vi "Log In.vi"(0 "session in":refnum<k21>, 1 "username":string, 2 "password":string, 5 "chassis":refnum<k21>, 11 "error in (no error)":errorcluster, 12 "connect timeout (60 sec)":dbl=60.0, 13 "save credentials to disk? (F)":bool) -> (4 "session out":refnum<k21>, 15 "error out":errorcluster)   [LabVIEW 2020, in "SLSC.lvlib"]
doc: "Saves login credentials for an SLSC chassis on the local system. When the SLSC driver opens a network connection to an SLSC chassis, it checks whether there are any saved login credentials for this chassis. If so, the SLSC driver uses the saved login credentials. Otherwise, the SLSC driver tries default credentials with anonymous as the username and an empty string as the password."
uses:
  <vilib>/SLSC/SLSC.lvlib
  nislsclvapi.dll
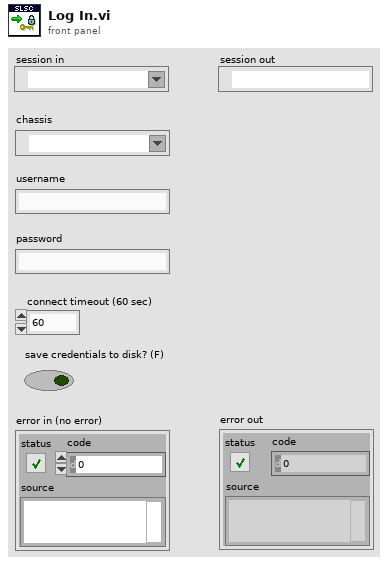
[diagram p1: front panel]
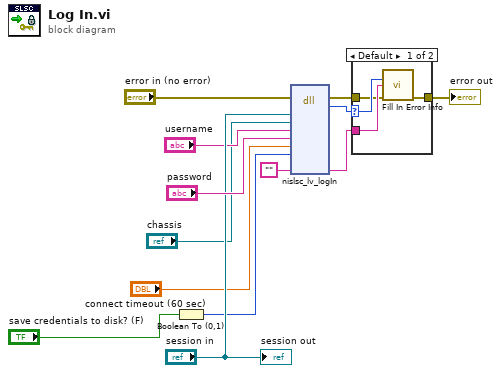
[diagram p0: block diagram]
diagram:
  n1 = Boolean To (0,1)(Boolean="save credentials to disk? (F)") -> (0, 1=w1:i16)
  n2 = dll-call lib="nislsclvapi.*" fn="nislsc_lv_logIn"(error in="error in (no error)", "session"="session in", "chassis"="chassis", "username"="username", "password"="password", "timeout"="connect timeout (60 sec)", "saveCredentialsToDisk"=w1, "extendedErrorInfo"="") -> (error out=w9:errorcluster, "return type"=w8:i32, "extendedErrorInfo"=w7:string)  [unwired: 10 in, 1 out]
  n3 = case shown="Default" w8 {
    selector: w8 -> [w17 _]
    tunnel: w7 -> [w16 _]
    tunnel: w9 -> [w15 w18]
    tunnel: [w14 w18] -> w6
    frame Default {
      n4 = call <vilib>:"Fill In Error Info.vi"("status code"=w17, "extended error info"=w16, "error in"=w15) -> ("error out"=w14:errorcluster)  [unwired: 12 in]
    }
    frame 0 {
    }
  }
  "error out" <- w6
  "session out" <- "session in"
